vi "Deserialize.vi"(8 "error in (no error)":errorcluster, 10 "String":string) -> (0 "error out":errorcluster, 3 "GameRecorder out":refnum<class "GameRecorder.lvclass">)   [LabVIEW 2015, in "TronviewGame.lvlib" / "GameRecorder.lvclass"]
uses:
  GameRecorder.lvclass
  TronVIEWBotAPI/MovementDirection.ctl
  GameRecorder.lvclass/GameRecorder.ctl
  Board/Board.lvclass
  TronVIEWBotAPI/TronVIEWBotAPI.lvlib
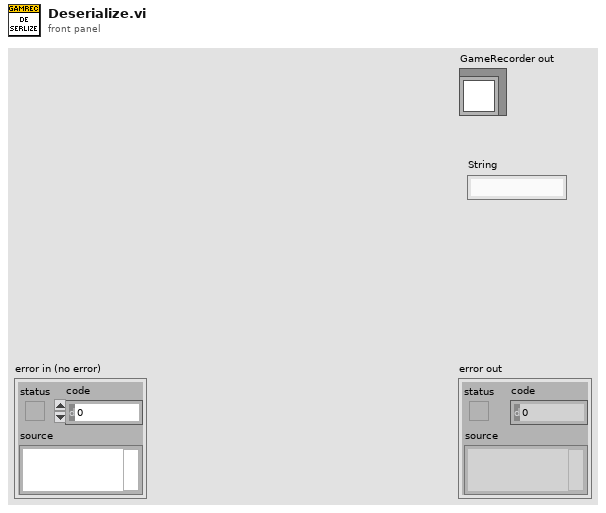
[diagram p1: front panel]
types:
  T1 = typedef "TronVIEWBotAPI.lvlib/MovementDirection.ctl" = enum16{"N", "S", "W", "E"}
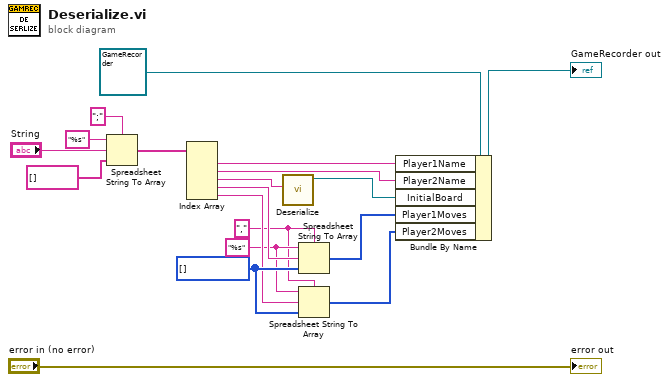
[diagram p0: block diagram]
diagram:
  w2 = "," ("delimiter (Tab)")
  w5 = T1[] [] items=["N", "S", "W", "E"] ("Player2Moves")
  w3 = "%s" ("format string")
  n1 = Spreadsheet String To Array(delimiter (Tab)=";", format string="%s", spreadsheet string="String", array type (2D Dbl)=string[] []) -> (array=w13:string[])
  n2 = Index Array(array=w13) -> (element #1=w11:string, element #2=w10:string, element #3=w9:string, element #4=w7:string, element #5=w4:string)  [unwired: 5 in]
  n3 = call "Deserialize.vi"("SerializedBoard"=w9) -> ("Board out"=w8:refnum<class "Board.lvclass">)  [unwired: 9 in, 1 out]
  n4 = Spreadsheet String To Array(delimiter (Tab)=w2, format string=w3, spreadsheet string=w7, array type (2D Dbl)=w5) -> (array=w6:T1[])
  n5 = Spreadsheet String To Array(delimiter (Tab)=w2, format string=w3, spreadsheet string=w4, array type (2D Dbl)=w5) -> (array=w1:T1[])
  n6 = Bundle By Name(cluster=refnum<class "GameRecorder.lvclass"> refnum ("GameRecorder in"), "Player1Name"=w11, "Player2Name"=w10, "InitialBoard"=w8, "Player1Moves"=w6, "Player2Moves"=w1) -> (→"GameRecorder out":refnum<class "GameRecorder.lvclass">)
  "error out" <- "error in (no error)"
